vi "Low-Pass Filter.vi"(7 "error in":errorcluster) -> (27 "error out":errorcluster)   [LabVIEW 2009]
uses:
  <vilib>/vision/NI_Vision_Development_Module.lvlib
panel:
  out "Image Out":T1(plugin-control)
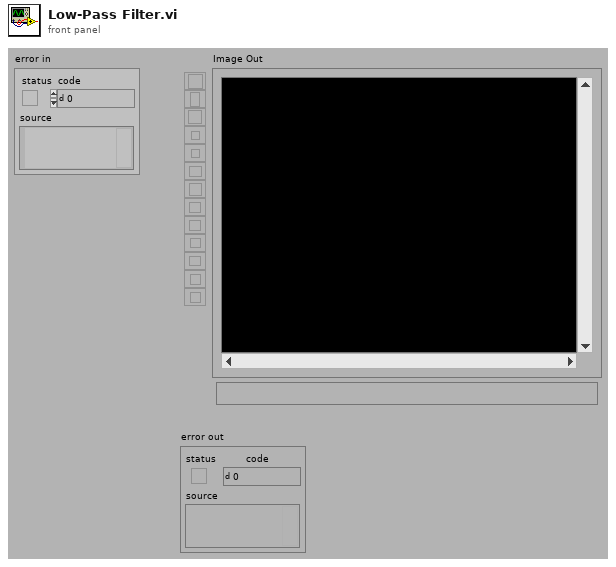
[diagram p1: front panel]
types:
  T1 = typedef "IMAQ Image.ctl" = refnum<image>
  T2 = cluster{"Measurement Parameter":i32, "Range Lower Value":dbl, "Range Upper Value":dbl, "Range":bool, "Measurement Type":bool}[]
  T3 = typedef "Image Type" = u32
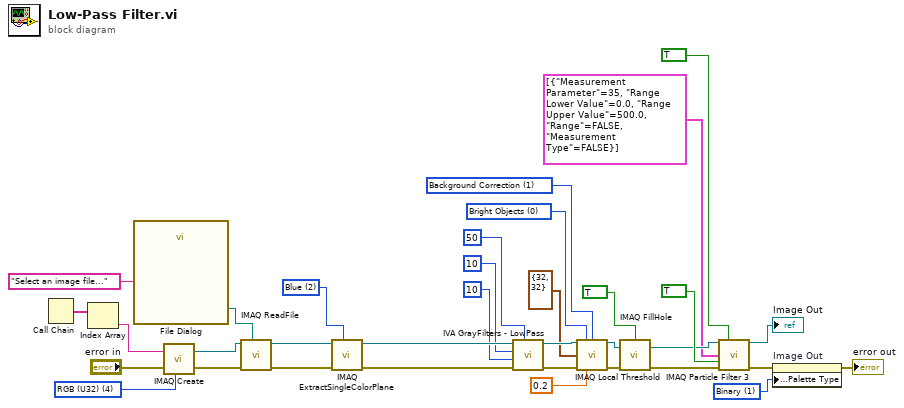
[diagram p0: block diagram]
diagram:
  w2 = u32 1 items=["Grayscale", "Binary", "Gradient", "Rainbow", "Temperature", "User Defined"] ("Palette")
  w13 = u32 0 items=["Bright Objects", "Dark Objects"] ("Look For (Bright Objects)")
  w16 = u32 1 items=["Niblack", "Background Correction"] ("Method")
  w25 = 2 items=["Red", "Green", "Blue", "Hue", "Saturation", "Luminance", "Value", "Intensity"] ("Color Plane")
  w26 = T3 4 items=["Grayscale (U8)", "Grayscale (I16)", "Grayscale (SGL)", "Complex (CSG)", "RGB (U32)", "HSL (U32)", "RGB (U64)", "Grayscale (U16)"] ("Image Type")
  n1 = Call Chain() -> (call chain=w30:string[])
  n2 = Index Array(array=w30) -> (element=w29:string)  [unwired: 1 in]
  n3 = call "File Dialog"("prompt"="Select an image file...") -> ("selected path"=w27:path)  [unwired: 6 in, 8 out]
  n4 = call "IMAQ Create"("Image Name"=w29, "Image Type"=w26, "error in (no error)"="error in") -> ("New Image"=w33:T1, "error out"=w32:errorcluster)  [unwired: 1 in, 1 out]
  n5 = call "IMAQ ReadFile"("File Path"=w27, "error in (no error)"=w32, "Image"=w33) -> ("error out"=w34:errorcluster, "Image Out"=w24:T1)  [unwired: 2 in, 5 out]
  n6 = call "IMAQ ExtractSingleColorPlane"("Color Plane"=w25, "error in (no error)"=w34, "Image Src"=w24) -> ("error out"=w23:errorcluster, "Image Dst Out"=w22:T1)  [unwired: 1 in, 6 out]
  n7 = call <vilib>:"IVA GrayFilters - LowPass.vi"("Tolerance"=50, "error in"=w23, "Filter size Y"=10, "Filter size X"=10, "Image In"=w22) -> ("error out"=w21:errorcluster, "Image Out"=w17:T1)  [unwired: 5 out]
  n8 = call "IMAQ Local Threshold"("Image Src"=w17, "Look For (Bright Objects)"=w13, "Method (Niblack)"=w16, "Window Size (32x32)"=cluster{"SizeX":i32, "SizeY":i32} {"SizeX"=32, "SizeY"=32} ("Kernel Size"), "error in (no error)"=w21, "Niblack Deviation Factor (0.2)"=0.2 ("Niblack Deviation Factor")) -> ("Image Dst Out"=w10:T1, "error out"=w12:errorcluster)  [unwired: 2 in, 6 out]
  n9 = call "IMAQ FillHole"("error in (no error)"=w12, "Image Src"=w10, "Connectivity 4/8 (8)"=TRUE) -> ("error out"=w9:errorcluster, "Image Dst Out"=w5:T1)  [unwired: 1 in, 2 out]
  n10 = call "IMAQ Particle Filter 3"("Image Src"=w5, "Connectivity 4/8 (8)"=TRUE, "Selection Values"=T2 [{"Measurement Parameter"=35, "Range Lower Value"=0.0, "Range Upper Value"=500.0, "Range"=FALSE, "Measurement Type"=FALSE}], "Keep/Remove Particles (F)"=TRUE ("Keep/Remove Particles"), "error in (no error)"=w9) -> ("Image Dst Out"=→"Image Out":T1, "error out"=w6:errorcluster)  [unwired: 4 in, 5 out]
  n11 = property on="Image Out" class="ImageControl"(error in=w6, "Palette:Palette Type"=w2) -> (error out=→"error out":errorcluster)  [unwired: 1 in, 1 out]
